vi "Storage Immediate Wrapper.vi"() -> ()   [LabVIEW 2019]
uses:
  Implementation/Storage Operations.ctl
panel:
  in  "Operation":T1
  in  "Spindexer Speed":dbl
  in  "Transfer Speed":dbl
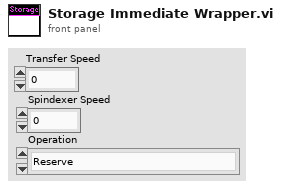
[diagram p1: front panel]
types:
  T1 = typedef "Storage Operations.ctl" = enum16{"Reserve", "Read Current", "Immediate", "Intake", "Shoot", "Override"}
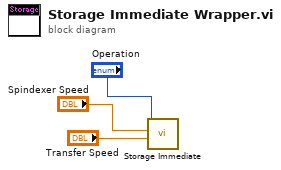
[diagram p0: block diagram]
diagram:
  n1 = call "Storage Immediate.vi"("Transfer Speed"="Transfer Speed", "Spindexer Speed"="Spindexer Speed", "Operation"="Operation") -> ()  [unwired: 9 in]
